vi "ReadInstrumentSettings.vi"(6 "Channels to scan (empty - don't use scanner option)":i32[](array[numeric]), 8 "error in (no error)":errorcluster, 9 "Initial String":string, 11 "Instrument type/address":T1={"Instrument"=enum."LkShr 340 chA&B", "VISA Resource"=""}) -> (0 "error out":errorcluster, 1 "Data titles":string[](array[string]), 2 "Parameters":string)   [LabVIEW 2015]
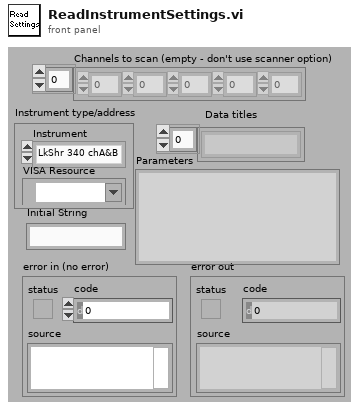
[diagram p1: front panel]
types:
  T1 = cluster{"Instrument":enum16{"NONE", "Neocera 21", "LakeShore 340", "LkShr 340 chA&B", "LakeShore 370", "SRS 850", "LR 700", "EG&G 5302", "EG&G 7260", "EG&G 7280", "AH 2500", "Keithley meter", "HP 5385", "HP 53181"}, "VISA Resource":refnum<visa-resource-name>}
  T2 = enum16{"NONE", "Neocera 21", "LakeShore 340", "LkShr 340 chA&B", "LakeShore 370", "SRS 850", "LR 700", "EG&G 5302", "EG&G 7260", "EG&G 7280", "AH 2500", "Keithley meter", "HP 5385", "HP 53181"}
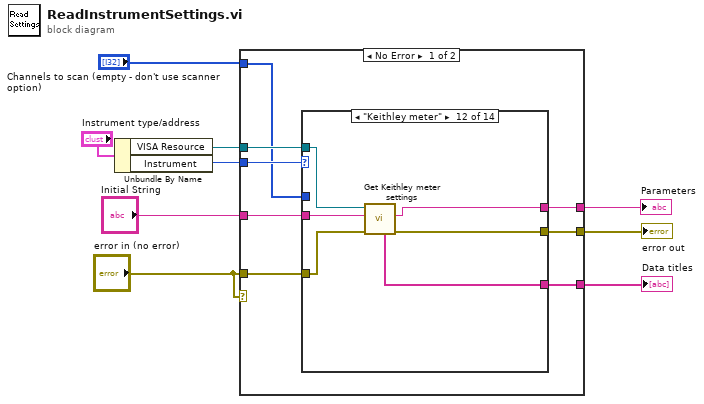
[diagram p0: block diagram]
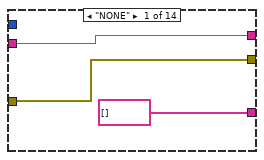
[diagram p2: hidden frame]
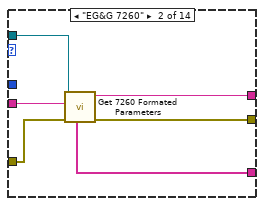
[diagram p3: hidden frame]
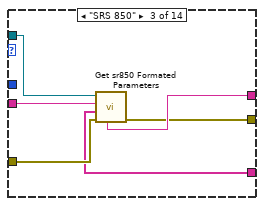
[diagram p4: hidden frame]
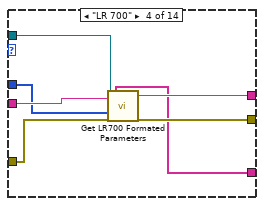
[diagram p5: hidden frame]
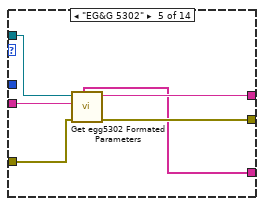
[diagram p6: hidden frame]
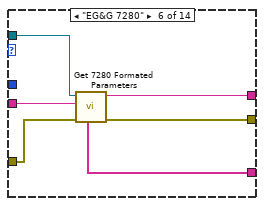
[diagram p7: hidden frame]
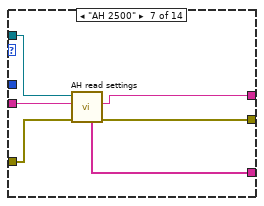
[diagram p8: hidden frame]
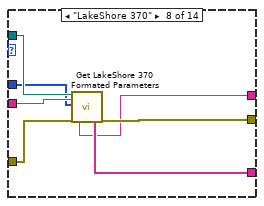
[diagram p9: hidden frame]
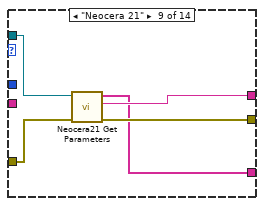
[diagram p10: hidden frame]
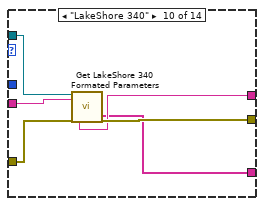
[diagram p11: hidden frame]
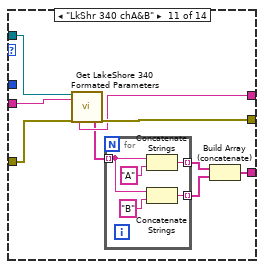
[diagram p12: hidden frame]
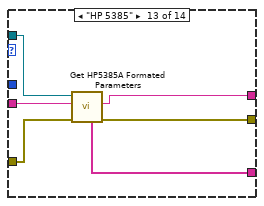
[diagram p13: hidden frame]
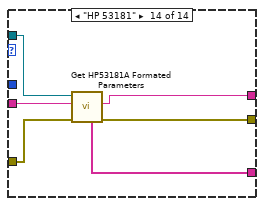
[diagram p14: hidden frame]
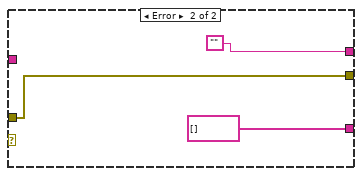
[diagram p15: hidden frame]
diagram:
  n1 = Unbundle By Name("Instrument type/address") -> ("VISA Resource"=w4:refnum<visa-resource-name>, "Instrument"=w3:T2)
  n2 = case shown="No Error" "error in (no error)" {
    tunnel: [w17 ""] -> w9
    tunnel: "Initial String" -> [w16 _]
    tunnel: "error in (no error)" -> [w15 w110]
    tunnel: [w14 w110] -> w7
    tunnel: [w11 string[] [] ("Data titles")] -> w6
    tunnel: w4 -> [w13 _]
    tunnel: w3 -> [w12 _]
    tunnel: "Channels to scan (empty - don't use scanner option)" -> [w10 _]
    frame No Error {
      n3 = case shown="\"Keithley meter\"" w12 {
        tunnel: w13 -> [_ w26 w32 w39 w45 w51 w54 w62 w66 w72 w81 w93 w99 w105]
        tunnel: [w19 w25 w31 w38 w41 w49 w55 w59 w67 w73 w82 w90 w96 w102] -> w17
        tunnel: w16 -> [w19 w24 w30 w37 w44 w47 w53 w61 _ w71 w80 w92 w98 w104]
        tunnel: w15 -> [w20 w23 w29 w36 w43 w50 w57 w64 w69 w75 w84 w95 w101 w107]
        tunnel: [w20 w22 w28 w35 w42 w48 w56 w63 w68 w74 w83 w94 w100 w106] -> w14
        tunnel: [string[] [] ("Data titles") w21 w27 w34 w40 w46 w52 w60 w65 w70 w78 w91 w97 w103] -> w11
        tunnel: w10 -> [_ _ _ w33 _ _ _ w58 _ _ _ _ _ _]
        frame "NONE" {
        }
        frame "EG&G 7260" {
          n4 = call "Get 7260 Formated Parameters.VI"("error in (no error)"=w23, "Initial String"=w24, "VISA Resource Name"=w26) -> ("error out"=w22:errorcluster, "Parameters"=w25:string, "Data titles"=w21:string[])  [unwired: 6 out]
        }
        frame "SRS 850" {
          n5 = call "Get sr850 Formated Parameters.VI"("error in (no error)"=w29, "Initial String"=w30, "VISA Resource Name"=w32) -> ("error out"=w28:errorcluster, "Parameters"=w31:string, "Data titles"=w27:string[])  [unwired: 6 out]
        }
        frame "LR 700" {
          n6 = call "Get LR700 Formated Parameters.vi"("VISA Resource Name"=w39, "Initial String"=w37, "Channels to scan (empty - don't use scanner option)"=w33, "error in (no error)"=w36) -> ("Data titles"=w34:string[], "Parameters"=w38:string, "error out"=w35:errorcluster)  [unwired: 13 out]
        }
        frame "EG&G 5302" {
          n7 = call "Get egg5302 Formated Parameters.VI"("error in (no error)"=w43, "Input String"=w44, "VISA Resource Name"=w45) -> ("error out"=w42:errorcluster, "Parameters"=w41:string, "Data titles"=w40:string[])  [unwired: 6 out]
        }
        frame "EG&G 7280" {
          n8 = call "Get 7280 Formated Parameters.VI"("error in (no error)"=w50, "Initial String"=w47, "VISA Resource Name"=w51) -> ("error out"=w48:errorcluster, "Parameters"=w49:string, "Data titles"=w46:string[])  [unwired: 6 out]
        }
        frame "AH 2500" {
          n9 = call "AH read settings.vi"("error in (no error)"=w57, "Initial string"=w53, "VISA Resource Name"=w54) -> ("error out"=w56:errorcluster, "Settings"=w55:string, "Data titles"=w52:string[])  [unwired: 6 out]
        }
        frame "LakeShore 370" {
          n10 = call "Get LakeShore 370 Formated Parameters.vi"("VISA Resource Name"=w62, "Initial String"=w61, "Channels to scan (empty - don't use scanner option)"=w58, "error in (no error)"=w64) -> ("Parameters"=w59:string, "Data titles"=w60:string[], "error out"=w63:errorcluster)  [unwired: 13 out]
        }
        frame "Neocera 21" {
          n11 = call "Neocera21 Get Parameters.vi"("error in (no error)"=w69, "VISA Resource Name"=w66) -> ("error out"=w68:errorcluster, "Parameters"=w67:string, "Data titles"=w65:string[])  [unwired: 1 in, 6 out]
        }
        frame "LakeShore 340" {
          n12 = call "Get LakeShore 340 Formated Parameters.vi"("VISA Resource Name"=w72, "Initial String"=w71, "error in (no error)"=w75) -> ("Parameters"=w73:string, "Data titles"=w70:string[], "error out"=w74:errorcluster)  [unwired: 14 out]
        }
        frame "LkShr 340 chA&B" {
          n13 = call "Get LakeShore 340 Formated Parameters.vi"("VISA Resource Name"=w81, "Initial String"=w80, "error in (no error)"=w84) -> ("Parameters"=w82:string, "Data titles"=w79:string[], "error out"=w83:errorcluster)  [unwired: 14 out]
          n14 = for {
            tunnel: w79 -> [w87] mode=indexing
            tunnel: [w86] -> w77 mode=indexing
            tunnel: [w85] -> w76 mode=indexing
            n15 = Concatenate Strings(w87, "A" ("string")) -> (w86:string)
            n16 = Concatenate Strings(w87, "B" ("string")) -> (w85:string)
          }
          n17 = Build Array (concatenate)(w77, w76) -> (w78:string[])
        }
        frame "Keithley meter" {
          n18 = call "Get Keithley meter settings.vi"("error in (no error)"=w95, "Initial string"=w92, "VISA Resource Name"=w93) -> ("error out"=w94:errorcluster, "Parameters"=w90:string, "Data titles"=w91:string[])  [unwired: 6 out]
        }
        frame "HP 5385" {
          n19 = call "Get HP5385A Formated Parameters.vi"("error in (no error)"=w101, "Initial String"=w98, "VISA Resource Name"=w99) -> ("error out"=w100:errorcluster, "Parameters"=w96:string, "Data titles"=w97:string[])  [unwired: 6 out]
        }
        frame "HP 53181" {
          n20 = call "Get HP53181A Formated Parameters.vi"("error in (no error)"=w107, "Initial String"=w104, "VISA Resource Name"=w105) -> ("error out"=w106:errorcluster, "Parameters"=w102:string, "Data titles"=w103:string[])  [unwired: 6 out]
        }
      }
    }
    frame Error {
    }
  }
  "error out" <- w7
  "Parameters" <- w9
  "Data titles" <- w6
